vi "pubKeyList.vi"(0 "HGF_GPG in":refnum<class "HGF_GPG.lvclass">, 1 "options file":path, 2 "keyringfile":path, 3 "Sec keyringfile":path, 5 "error in (no error)":errorcluster, 6 "Trust DB":path) -> (12 "dup Trust DB":path, 14 "HGF_GPG out":refnum<class "HGF_GPG.lvclass">, 15 "dup options file":path, 16 "dup keyringfile":path, 17 "dup Sec keyringfile":path, 18 "pub keys":string[](array[string]), 19 "error out":errorcluster)   [LabVIEW 2012, in "HGF_GPG.lvlib" / "HGF_GPG.lvclass"]
doc: "returns a list of all the keys stored in public keyring file\n\nF.Berck@gsi.de"
uses:
  HGF_GPG.lvclass
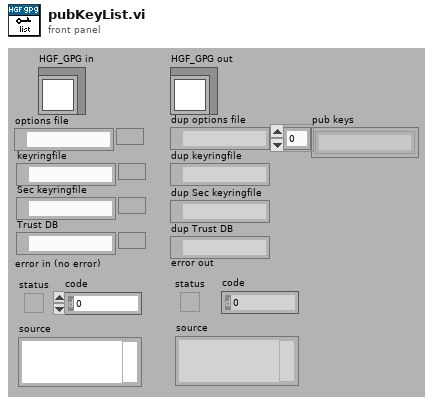
[diagram p1: front panel]
types:
  T1 = enum16{"list keys", "export", "import", "delete"}
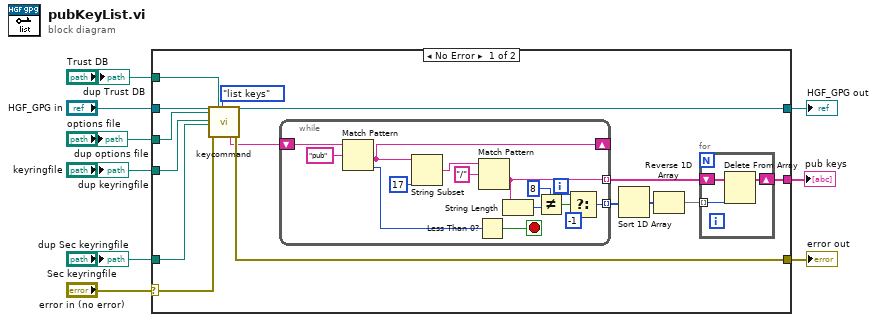
[diagram p0: block diagram]
diagram:
  n1 = case shown="No Error" "error in (no error)" {
    selector: "error in (no error)" -> [w19 w44]
    tunnel: [w16 w44] -> w8
    tunnel: [w23 w43] -> w6
    tunnel: "HGF_GPG in" -> [w24 w43]
    tunnel: "options file" -> [w22 _]
    tunnel: "keyringfile" -> [w21 _]
    tunnel: "Sec keyringfile" -> [w20 _]
    tunnel: "Trust DB" -> [w18 _]
    tunnel: [w10 _] -> w1
    frame No Error {
      n2 = call-dynamic "keycommand.vi"("HGF_GPG in"=w24, "options file"=w22, "keyringfile"=w21, "Sec keyringfile"=w20, "error in (no error)"=w19, "Trust DB"=w18, "Enum"=T1."list keys") -> ("standard output"=w15:string, "HGF_GPG out"=w23:refnum<class "HGF_GPG.lvclass">, "error out"=w16:errorcluster)  [unwired: 4 in, 14 out]
      n3 = while {
        shift-right: [w37] -> _
        shift-left: w15 -> [w42]
        tunnel: [w34] -> w12 mode=indexing
        tunnel: [w28] -> w13 mode=indexing
        i -> [w30]
        stop <- w39 stop-if-true
        n4 = Match Pattern(string=w42, regular expression="pub") -> (after substring=w37:string, offset past match=w41:i32)  [unwired: 3 out]
        n5 = String Subset(string=w37, length (rest)=17 ("length (rest)")) -> (substring=w36:string)  [unwired: 1 out]
        n6 = Less Than 0?(x=w41) -> (x < 0?=w39:bool)
        n7 = Match Pattern(string=w36, regular expression="/") -> (after substring=w34:string)  [unwired: 4 out]
        n8 = String Length(string=w34) -> (length=w33:i32)
        n9 = Not Equal?(x=w33, y=8) -> (x != y?=w31:bool)
        n10 = Select(t=w30, s=w31, f=-1) -> (s? t:f=w28:i32)
      }
      n11 = Sort 1D Array(array=w13) -> (sorted array=w14:i32[])
      n12 = Reverse 1D Array(array=w14) -> (reversed array=w11:i32[])
      n13 = for {
        tunnel: w11 -> [w27] mode=indexing
        shift-right: [w25] -> w10
        shift-left: w12 -> [w26]
        n14 = Delete From Array(array=w26, index=w27) -> (array with subset deleted=w25:string[])  [unwired: 1 in, 1 out]
      }
    }
    frame Error {
    }
  }
  "error out" <- w8
  "HGF_GPG out" <- w6
  "pub keys" <- w1
  "dup Trust DB" <- "Trust DB"
  "dup options file" <- "options file"
  "dup keyringfile" <- "keyringfile"
  "dup Sec keyringfile" <- "Sec keyringfile"
